vi "Load CSV File.vi"(8 "error in (no error)":errorcluster, 10 "Channel":string, 11 "selected path":path) -> (0 "error out":errorcluster, 2 "LUT":variant, 3 "path":path)   [LabVIEW 2013, in "OPC UA Client System Explorer.lvlib"]
uses:
  OPC UA Client System Explorer.lvlib
  <vilib>/Utility/miscctls.llb/LVStringsAndValuesArrayTypeDef_U32.ctl
  Types/Tag.Settings
  <userlib>/_OpenG.lib/array/array.llb/Sort 2D Array (String)__ogtk.vi
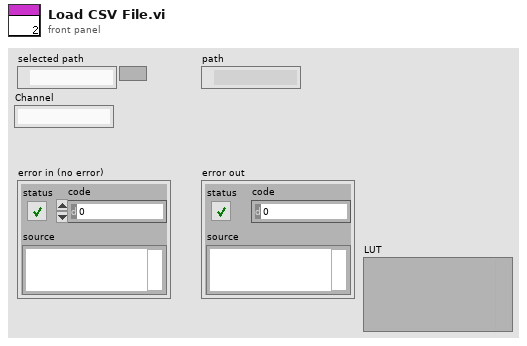
[diagram p1: front panel]
types:
  T1 = typedef "LVStringsAndValuesArrayTypeDef_U32.ctl" = cluster{"String":string, "Value":u32}[]
  T2 = enum16{"open", "replace", "create", "open or create", "replace or create", "replace or create with confirmation"}
  T3 = typedef "Tag.Settings" = cluster{"Settings":cluster{"name":string, "node type":enum32{"Other", "Folder", "Item/Property"}, "DataType":u32, "access":enum16{"Null", "Read", "Write", "Read&Write"}, "description":string}, "Array Size":i32}
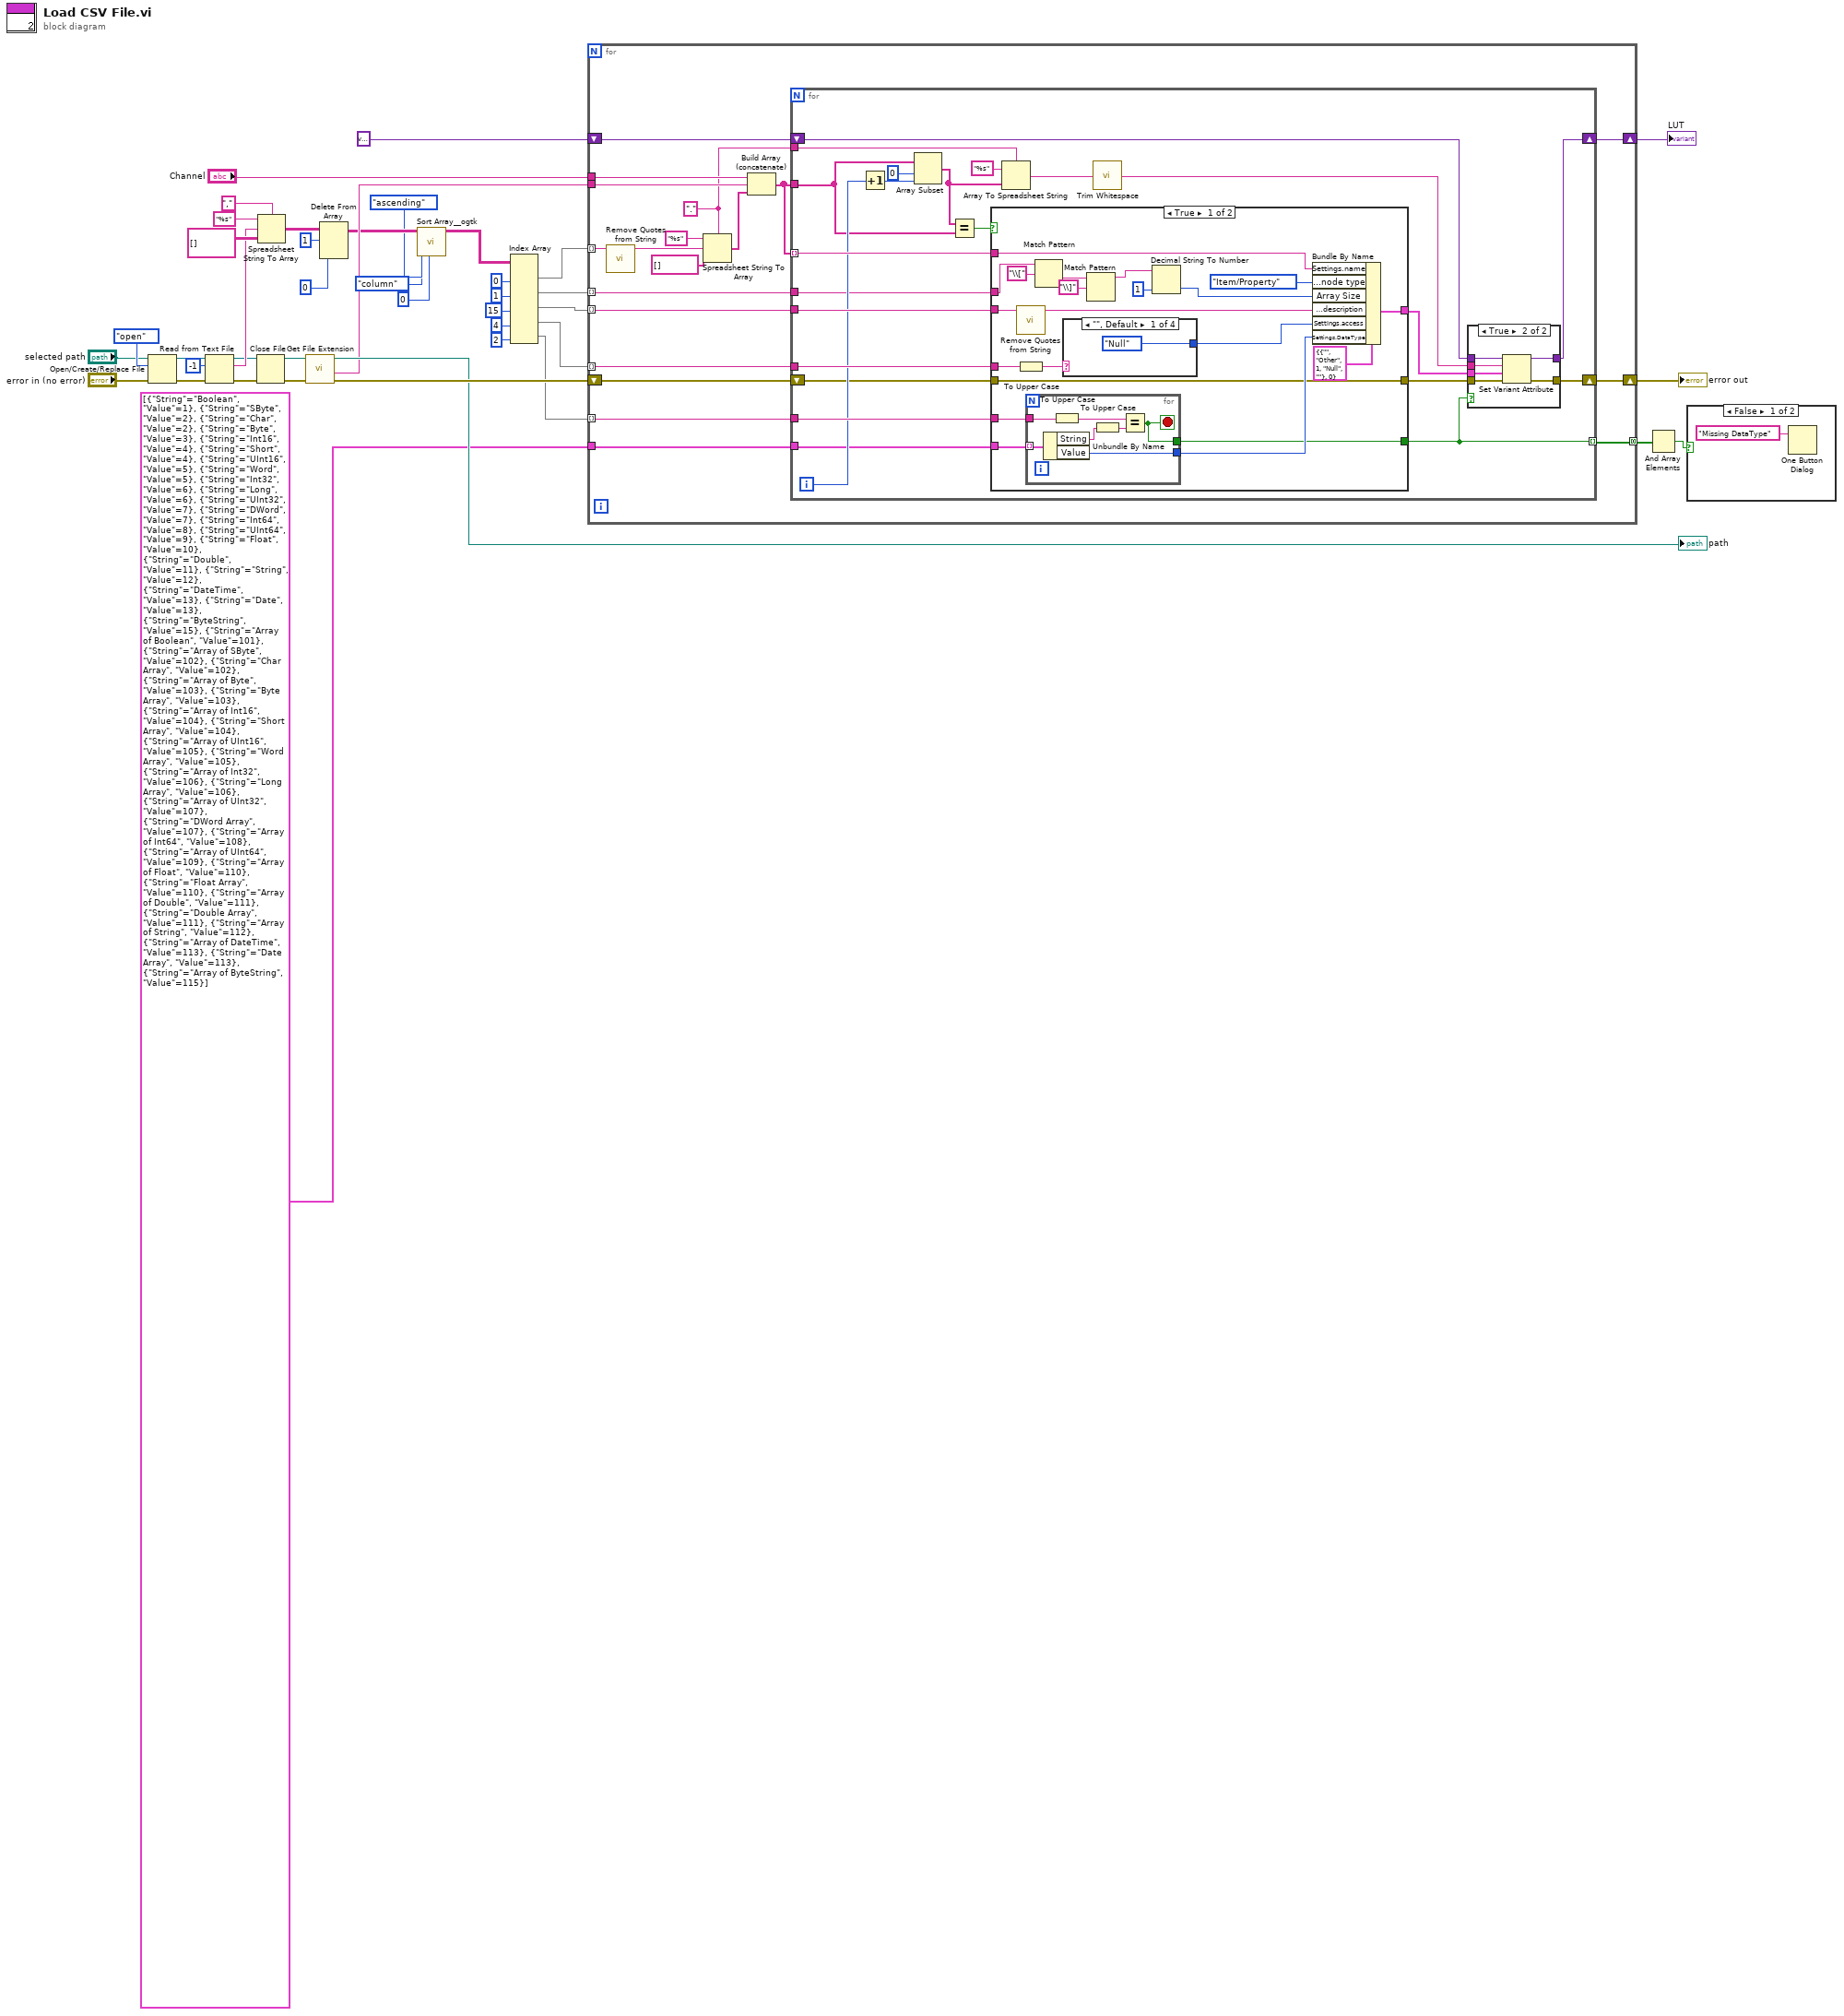
[diagram p0: block diagram]
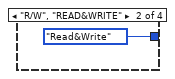
[diagram p4: hidden frame]
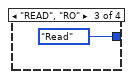
[diagram p5: hidden frame]
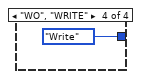
[diagram p6: hidden frame]
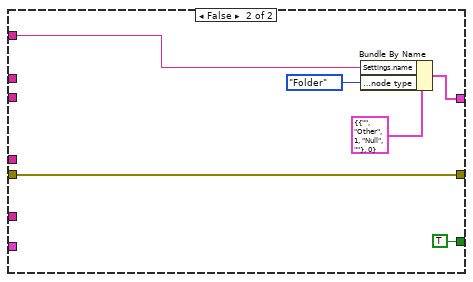
[diagram p7: hidden frame]
diagram:
  n1 = Open/Create/Replace File(file path (use dialog)="selected path", error in="error in (no error)", operation (0:open)=T2."open") -> (refnum out=w34:refnum<file>, error out=w31:errorcluster)  [unwired: 3 in, 1 out]
  n2 = Read from Text File(file (use dialog)=w34, count=-1, error in=w31) -> (refnum out=w33:refnum<file>, text=w38:string, error out=w32:errorcluster)  [unwired: 1 in, 1 out]
  n3 = Close File(refnum=w33, error in=w32) -> (path=w22:path, error out=w24:errorcluster)
  n4 = Spreadsheet String To Array(delimiter (Tab)=",", format string="%s", spreadsheet string=w38, array type (2D Dbl)=string[][] []) -> (array=w28:string[][])
  n5 = call <vilib>:"Get File Extension.vi"("error in (no error)"=w24, "file"=w22) -> ("error out"=w23:errorcluster, "filename without extension"=w19:string, "dup file"=→"path":path)  [unwired: 6 in, 1 out]
  n6 = Delete From Array(array=w28, length=1, index (row)=0) -> (array with subset deleted=w15:string[][])  [unwired: 1 in, 1 out]
  n7 = call-poly <userlib>:"Sort Array__ogtk.vi"("Column/Row to Sort By"=u32 0, "Sort By in"=enum16{"row", "column"}."column", "Order"=enum16{"ascending", "descending"}."ascending", "Array in"=w15) -> ("Sorted Array out"=w14:string[][])  [unwired: 4 in, 3 out]
  n8 = Index Array(array=w14, index (col) #1=0 ("disabled index (col)"), index (col) #2=1 ("index (col)"), index (col) #3=15 ("index (col)"), index (col) #4=4 ("index (col)"), index (col) #5=2 ("index (col)")) -> (element #1=w29:string[], element #2=w3:string[], element #3=w5:string[], element #4=w7:string[], element #5=w9:string[])  [unwired: 5 in]
  n9 = for {
    tunnel: w9 -> [w59] mode=indexing
    tunnel: w7 -> [w60] mode=indexing
    tunnel: w5 -> [w61] mode=indexing
    tunnel: w29 -> [w46] mode=indexing
    shift-right: [w54] -> w17
    shift-left: w23 -> [w52]
    shift-right: [w55] -> w18
    shift-left: variant ("variant") -> [w57]
    tunnel: "Channel" -> [w58]
    tunnel: w19 -> [w53]
    tunnel: T1 [{"String"="Boolean", "Value"=1}, {"String"="SByte", "Value"=2}, {"String"="Char", "Value"=2}, {"String"="Byte", "Value"=3}, {"String"="Int16", "Value"=4}, {"String"="Short", "Value"=4}, {"String"="UInt16", "Value"=5}, {"String"="Word", "Value"=5}, {"String"="Int32", "Value"=6}, {"String"="Long", "Value"=6}, {"String"="UInt32", "Value"=7}, {"String"="DWord", "Value"=7}, {"String"="Int64", "Value"=8}, {"String"="UInt64", "Value"=9}, {"String"="Float", "Value"=10}, {"String"="Double", "Value"=11}, {"String"="String", "Value"=12}, {"String"="DateTime", "Value"=13}, {"String"="Date", "Value"=13}, {"String"="ByteString", "Value"=15}, {"String"="Array of Boolean", "Value"=101}, {"String"="Array of SByte", "Value"=102}, {"String"="Char Array", "Value"=102}, {"String"="Array of Byte", "Value"=103}, {"String"="Byte Array", "Value"=103}, {"String"="Array of Int16", "Value"=104}, {"String"="Short Array", "Value"=104}, {"String"="Array of UInt16", "Value"=105}, {"String"="Word Array", "Value"=105}, {"String"="Array of Int32", "Value"=106}, {"String"="Long Array", "Value"=106}, {"String"="Array of UInt32", "Value"=107}, {"String"="DWord Array", "Value"=107}, {"String"="Array of Int64", "Value"=108}, {"String"="Array of UInt64", "Value"=109}, {"String"="Array of Float", "Value"=110}, {"String"="Float Array", "Value"=110}, {"String"="Array of Double", "Value"=111}, {"String"="Double Array", "Value"=111}, {"String"="Array of String", "Value"=112}, {"String"="Array of DateTime", "Value"=113}, {"String"="Date Array", "Value"=113}, {"String"="Array of ByteString", "Value"=115}] ("Strings And Values []") -> [w47]
    tunnel: w3 -> [w44] mode=indexing
    tunnel: [w43] -> w2 mode=concatenating
    w49 = "." ("delimiter (Tab)")
    n10 = call "Remove Quotes from String.vi"("String in"=w46) -> ("String out"=w45:string)  [unwired: 10 in]
    n11 = Spreadsheet String To Array(delimiter (Tab)=w49, format string="%s" ("spreadsheet string"), spreadsheet string=w45, array type (2D Dbl)=string[] []) -> (array=w51:string[])
    n12 = Build Array (concatenate)(w58, w53, w51) -> (w56:string[])
    n13 = for {
      tunnel: w56 -> [w81] mode=indexing
      tunnel: w61 -> [w84]
      tunnel: w60 -> [w83]
      tunnel: w59 -> [w82]
      tunnel: w56 -> [w74]
      shift-right: [w77] -> w54
      shift-left: w52 -> [w65]
      shift-right: [w72] -> w55
      shift-left: w57 -> [w76]
      tunnel: w49 -> [w69]
      tunnel: w47 -> [w67]
      tunnel: w44 -> [w63]
      tunnel: [w62] -> w43 mode=indexing
      i -> [w78]
      n14 = Increment(x=w78) -> (x+1=w79:i32)
      n15 = Array Subset(array=w74, index=0, length=w79) -> (w71:string[])
      n16 = Equal?(x=w71, y=w74) -> (x = y?=w73:bool)
      n17 = case shown="True" w73 {
        tunnel: w84 -> [w105 _]
        tunnel: w83 -> [w112 _]
        tunnel: w82 -> [w109 _]
        tunnel: w81 -> [w107 w129]
        tunnel: [w102 w128] -> w75
        tunnel: w67 -> [w106 _]
        tunnel: w65 -> [w104 w127]
        tunnel: [w104 w127] -> w64
        tunnel: w63 -> [w100 _]
        tunnel: [w93 TRUE] -> w62
        frame True {
          n18 = call "Remove Quotes from String.vi"("String in"=w105) -> ("String out"=w101:string)  [unwired: 10 in]
          n19 = To Upper Case(1:w112) -> (0:w110:string)
          n20 = for {
            tunnel: w106 -> [w120] mode=indexing
            tunnel: w109 -> [w118]
            tunnel: [w115] -> w108
            tunnel: [w114] -> w93
            stop <- w114 stop-if-true
            n21 = Unbundle By Name(w120) -> ("String"=w119:string, "Value"=w115:u32)
            n22 = To Upper Case(1:w118) -> (0:w117:string)
            n23 = To Upper Case(1:w119) -> (0:w116:string)
            n24 = Equal?(x=w117, y=w116) -> (x = y?=w114:bool)
          }
          n25 = Match Pattern(string=w100, regular expression="\\[") -> (after substring=w98:string)  [unwired: 1 in, 3 out]
          n26 = case shown="\"\", Default" w110 {
            tunnel: [enum16{"Null", "Read", "Write", "Read&Write"}."Null" ("access") enum16{"Null", "Read", "Write", "Read&Write"}."Read&Write" ("access") enum16{"Null", "Read", "Write", "Read&Write"}."Read" ("access") enum16{"Null", "Read", "Write", "Read&Write"}."Write" ("access")] -> w111
            frame "", Default {
            }
            frame "R/W", "READ&WRITE" {
            }
            frame "READ", "RO" {
            }
            frame "WO", "WRITE" {
            }
          }
          n27 = Match Pattern(string=w98, regular expression="\\]") -> (before substring=w96:string)  [unwired: 1 in, 3 out]
          n28 = Decimal String To Number(string=w96, default (0L)=1 ("default (0 I32)")) -> (number=w94:i32)  [unwired: 1 in, 1 out]
          n29 = Bundle By Name(cluster=T3 {"Settings"={"name"="", "node type"=enum."Other", "DataType"=1, "access"=enum."Null", "description"=""}, "Array Size"=0}, "Settings.name"=w107, "Settings.node type"=enum32{"Other", "Folder", "Item/Property"}."Item/Property" ("node type"), "Array Size"=w94, "Settings.description"=w101, "Settings.access"=w111, "Settings.DataType"=w108) -> (w102:T3)
        }
        frame False {
          n30 = Bundle By Name(cluster=T3 {"Settings"={"name"="", "node type"=enum."Other", "DataType"=1, "access"=enum."Null", "description"=""}, "Array Size"=0}, "Settings.name"=w129, "Settings.node type"=enum32{"Other", "Folder", "Item/Property"}."Folder" ("node type")) -> (w128:T3)
        }
      }
      n31 = Array To Spreadsheet String(delimiter (Tab)=w69, array=w71, 3:"%s" ("format string")) -> (spreadsheet string=w70:string)
      n32 = call <vilib>:"Trim Whitespace.vi"("string"=w70) -> ("trimmed string"=w66:string)  [unwired: 1 in]
      n33 = case shown="True" w62 {
        tunnel: [w86 w92] -> w77
        tunnel: w76 -> [w85 w91]
        tunnel: w75 -> [_ w90]
        tunnel: [w85 w89] -> w72
        tunnel: w66 -> [_ w88]
        tunnel: w64 -> [w86 w87]
        frame False {
        }
        frame True {
          n34 = Set Variant Attribute(Variant=w91, name=w88, value=w90, error in=w87) -> (Variant out=w89:variant, error out=w92:errorcluster)  [unwired: 1 out]
        }
      }
    }
  }
  "error out" <- w17
  "LUT" <- w18
  n35 = And Array Elements(Boolean array=w2) -> (logical AND=w1:bool)
  n36 = case shown="False" w1 {
    frame False {
      n37 = One Button Dialog(message="Missing DataType") -> ()  [unwired: 1 in, 1 out]
    }
    frame True {
    }
  }
